vi "Solve Complex Linear Equations.vi"   [LabVIEW 2010, in "NI_AALBase.lvlib"]
doc: "Solves a complex linear system AX=Y."
uses:
  NI_AALBase.lvlib
  NI_AALPro.lvlib
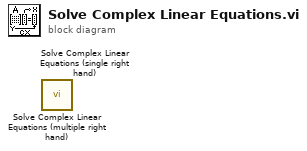
[diagram p0: block diagram]
diagram:
  n1 = call "Solve Complex Linear Equations (multiple right hand).vi"() -> ()  [unwired: 3 in, 2 out]
  n2 = call "Solve Complex Linear Equations (single right hand).vi"() -> ()  [unwired: 3 in, 2 out]
